vi "DiffDrvOdom2_Execute.vi"(6 "Initial Pose Meters":T1={"TRANSLATION"={"X"=0.0, "Y"=0.0}, "ROTATION"={"VALUE"=0.0, "COS"=1.0, "SIN"=0.0}} {"ROTATION"."SIN" format="%13.4f"; "ROTATION"."COS" format="%13.4f"; "ROTATION"."VALUE" format="%13.4f"; "TRANSLATION"."Y" format="%14.3f"; "TRANSLATION"."X" format="%14.3f"}, 8 "Init / Reset":bool, 9 "Right Distance M":dbl, 10 "Left Distance M":dbl, 11 "Gyro Reading":T3={"VALUE"=0.0, "COS"=1.0, "SIN"=0.0} {"SIN" format="%13.4f"; "COS" format="%13.4f"; "VALUE" format="%13.4f"}) -> (1 "Pose Meters":T1={"TRANSLATION"={"X"=0.0, "Y"=0.0}, "ROTATION"={"VALUE"=0.0, "COS"=1.0, "SIN"=0.0}} {"ROTATION"."SIN" format="%13.4f"; "ROTATION"."COS" format="%13.4f"; "ROTATION"."VALUE" format="%13.4f"; "TRANSLATION"."Y" format="%14.3f"; "TRANSLATION"."X" format="%14.3f"}, 3 "Out DIFF_DRIVE_ODOM":T4={"M_POSE_Meters"={"TRANSLATION"={"X"=0.0, "Y"=0.0}, "ROTATION"={"VALUE"=0.0, "COS"=1.0, "SIN"=0.0}}, "M_GyroOffset"={"VALUE"=0.0, "COS"=1.0, "SIN"=0.0}, "M_PrevAngle"={"VALUE"=0.0, "COS"=1.0, "SIN"=0.0}, "M_PrevLeftDist_M"=0.0, "M_PrevRightDist_M"=0.0, "M_InitLeftDist_M"=0.0, "M_InitRightDist_M"=0.0} {"M_PrevAngle"."SIN" format="%13.4f"; "M_PrevAngle"."COS" format="%13.4f"; "M_PrevAngle"."VALUE" format="%13.4f"; "M_GyroOffset"."SIN" format="%13.4f"; "M_GyroOffset"."COS" format="%13.4f"; "M_GyroOffset"."VALUE" format="%13.4f"; "M_POSE_Meters"."ROTATION"."SIN" format="%13.4f"; "M_POSE_Meters"."ROTATION"."COS" format="%13.4f"; "M_POSE_Meters"."ROTATION"."VALUE" format="%13.4f"; "M_POSE_Meters"."TRANSLATION"."Y" format="%14.3f"; "M_POSE_Meters"."TRANSLATION"."X" format="%14.3f"})   [LabVIEW 2019, in "Trajectory_Library.lvlib"]
doc: "Single call LabVIEW VI to perform differential drive odometry. Odometry allows you to track the robot's position on the field over the course of a match using readings from 2 encoders and a gyroscope.\n \nTeams can use odometry during the autonomous period for complex tasks like path following. Furthermore, odometry can be used for latency compensation when using computer-vision systems.\n\nUpdates the robot position on the field using distance measurements from encoders. This method is more numerically accurate than using velocities to integrate the pose and is also advantageous for teams that are using lower CPR encoders.\n\n\nInputs:\n - gyroAngle -- Rotation2d -- The angle reported by the gyroscope.\n - leftDistanceMeters -- double -- The distance traveled by the left encoder.\n - rightDistanceMeters -- double -- The distance traveled by the right encoder.\n - init/reset -- boolean -- When TRUE, position, gyro, and distances are reset.\n - initialPoseMeters -- Pose2d -- The starting position of the robot on the field.\n\nOutputs:\n - out_DiffDriveOdom -- DiffDriveOdom2 -- Current value of internal data cluster\n -- Pose meters -- Pose2d -- Current robot location.\n\n\n\n \nInputs:\n - in_DiffDriveOdom -- DiffDriveOdom2 -- Diff Drive odometry data cluster\n - gyroAngle The angle reported by the gyroscope.\n - leftDistanceMeters The distance traveled by the left encoder.\n - rightDistanceMeters The distance traveled by the right encoder.\n\nOutputs:\n - out_DiffDriveOdom -- DiffDriveOdom2 -- Updated data cluster\n - pose -- Pose2d -- The new pose of the robot."
uses:
  TypeDef/DIFF_DRIVE_ODOM2.ctl
  TypeDef/POSE2D.ctl
  TypeDef/TRANSLATION2D.ctl
  TypeDef/ROTATION2D.ctl
  Rotation2d_UnaryMinus.vi
  Rotation2d_RotateBy.vi
  Rotation2d_CreateAngle.vi
  Rotation2d_CreateXY.vi
  Util_CalcDist.vi
  Trajectory_Library.lvlib
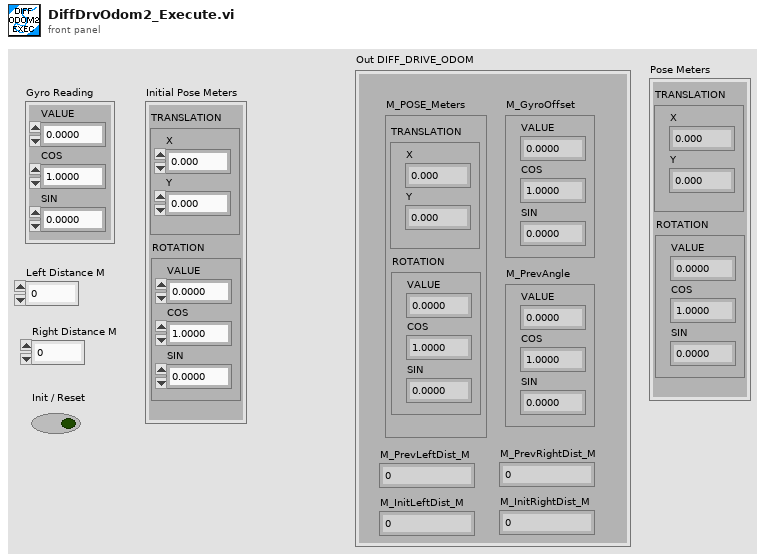
[diagram p1: front panel]
types:
  T1 = typedef "Trajectory_Library.lvlib/POSE2D.ctl" = cluster{"TRANSLATION":T2, "ROTATION":T3}
  T2 = typedef "Trajectory_Library.lvlib/TRANSLATION2D.ctl" = cluster{"X":dbl, "Y":dbl}
  T3 = typedef "Trajectory_Library.lvlib/ROTATION2D.ctl" = cluster{"VALUE":dbl, "COS":dbl, "SIN":dbl}
  T4 = typedef "Trajectory_Library.lvlib/DIFF_DRIVE_ODOM2.ctl" = cluster{"M_POSE_Meters":T1, "M_GyroOffset":T3, "M_PrevAngle":T3, "M_PrevLeftDist_M":dbl, "M_PrevRightDist_M":dbl, "M_InitLeftDist_M":dbl, "M_InitRightDist_M":dbl}
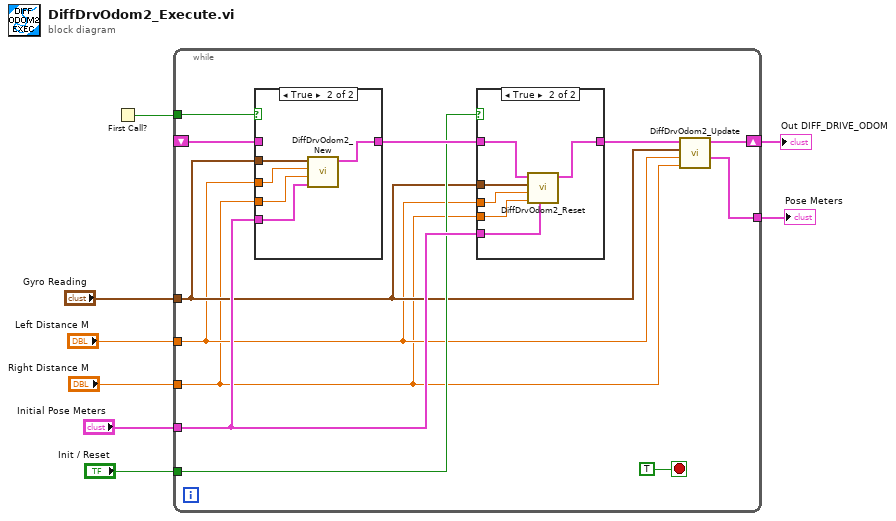
[diagram p0: block diagram]
diagram:
  n1 = First Call?() -> (First Call?: T/F=w8:bool)
  n2 = while {
    tunnel: w8 -> [w19]
    tunnel: "Gyro Reading" -> [w11]
    tunnel: "Left Distance M" -> [w10]
    tunnel: "Right Distance M" -> [w9]
    tunnel: "Initial Pose Meters" -> [w13]
    shift-right: [w15] -> w3
    shift-left: _ -> [w18]
    tunnel: [w14] -> w2
    tunnel: "Init / Reset" -> [w12]
    stop <- TRUE stop-if-true
    n3 = case shown="True" w19 {
      tunnel: w11 -> [_ w33]
      tunnel: w10 -> [_ w32]
      tunnel: w9 -> [_ w31]
      tunnel: w13 -> [_ w30]
      tunnel: [w28 w29] -> w17
      tunnel: w18 -> [w28 _]
      frame False {
      }
      frame True {
        n4 = call "DiffDrvOdom2_New.vi"("Initial Pose Meters"=w30, "Initial Right Distance M"=w31, "Initial Left Distance M"=w32, "Initial Gyro Reading"=w33) -> ("Out DIFF_DRIVE_ODOM"=w29:T4)  [unwired: 7 in]
      }
    }
    n5 = case shown="True" w12 {
      tunnel: [w21 w27] -> w16
      tunnel: w17 -> [w21 w26]
      tunnel: w11 -> [_ w25]
      tunnel: w10 -> [_ w24]
      tunnel: w9 -> [_ w23]
      tunnel: w13 -> [_ w22]
      frame False {
      }
      frame True {
        n6 = call "DiffDrvOdom2_Reset.vi"("Pose Meters"=w22, "Right Distance M"=w23, "Left Distance M"=w24, "Gyro Reading"=w25, "In DIFF_DRIVE_ODOM"=w26) -> ("Out DIFF_DRIVE_ODOM"=w27:T4)  [unwired: 6 in]
      }
    }
    n7 = call "DiffDrvOdom2_Update.vi"("Right Distance M"=w9, "Left Distance M"=w10, "Gyro Reading"=w11, "In DIFF_DRIVE_ODOM"=w16) -> ("Pose Meters"=w14:T1, "Out DIFF_DRIVE_ODOM"=w15:T4)  [unwired: 6 in]
  }
  "Out DIFF_DRIVE_ODOM" <- w3
  "Pose Meters" <- w2
